vi "close.vi"(8 "error in":errorcluster, 11 "module in":refnum<class "Watchdog runtime.lvclass">) -> (0 "error out":errorcluster)   [LabVIEW 2013, in "Watchdog runtime.lvclass"]
doc: "Provides an interface for terminating a module instance. While this interface performs no operations, a child should close and deallocate any open references or memory."
uses:
  Watchdog runtime.lvclass
  <vilib>/NI/DCAF/Tag Editor Core/control module/runtime/control module runtime.lvclass
  Watchdog runtime.lvclass/Watchdog runtime.ctl
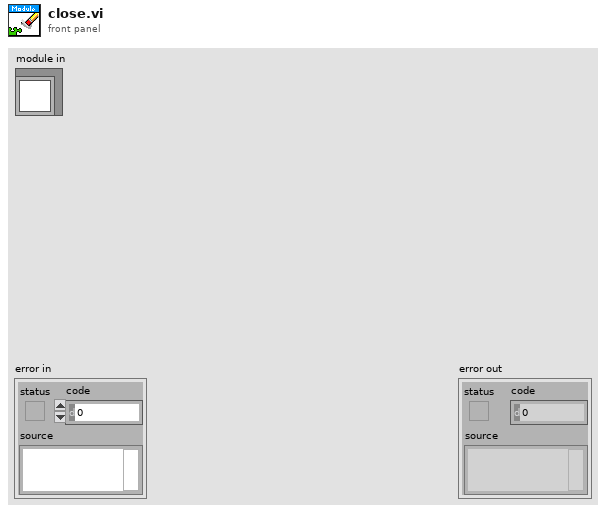
[diagram p1: front panel]
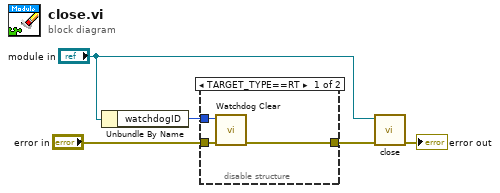
[diagram p0: block diagram]
diagram:
  n1 = Unbundle By Name("module in") -> ("watchdogID"=w3:u32)
  n2 = disable-structure shown="TARGET_TYPE==RT" {
    disable-tunnel: w3 -> [w8 _]
    disable-tunnel: [w7 w9] -> w2
    disable-tunnel: "error in" -> [w6 w9]
    frame condition #0 (active) {
      n3 = call <vilib>:"Watchdog Clear.vi"("error in (no error)"=w6, "watchdogID in"=w8) -> ("error out"=w7:errorcluster)  [unwired: 5 in]
    }
    frame condition #1 {
    }
  }
  n4 = call-parent "close.vi"("error in"=w2, "module in"="module in") -> ("error out"=→"error out":errorcluster)  [unwired: 9 in]
